vi "GetConfigure.vi"(8 "Error In":errorcluster, 11 "Keithley 6482 In":refnum<visa-resource-name>) -> (0 "Error Out":errorcluster, 2 "Configuration":string, 3 "Keithley 6482 Out":refnum<visa-resource-name>)   [LabVIEW 2014, in "Keithley-6482-Visa.lvlib"]
uses:
  Keithley-6482-Visa.lvlib
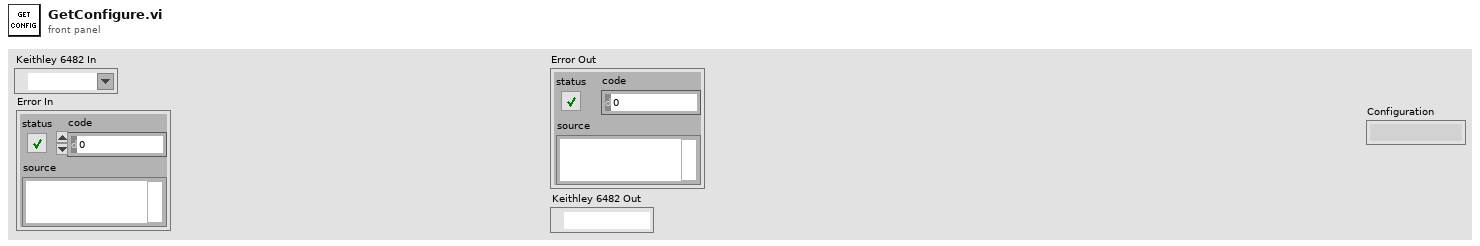
[diagram p1: front panel]
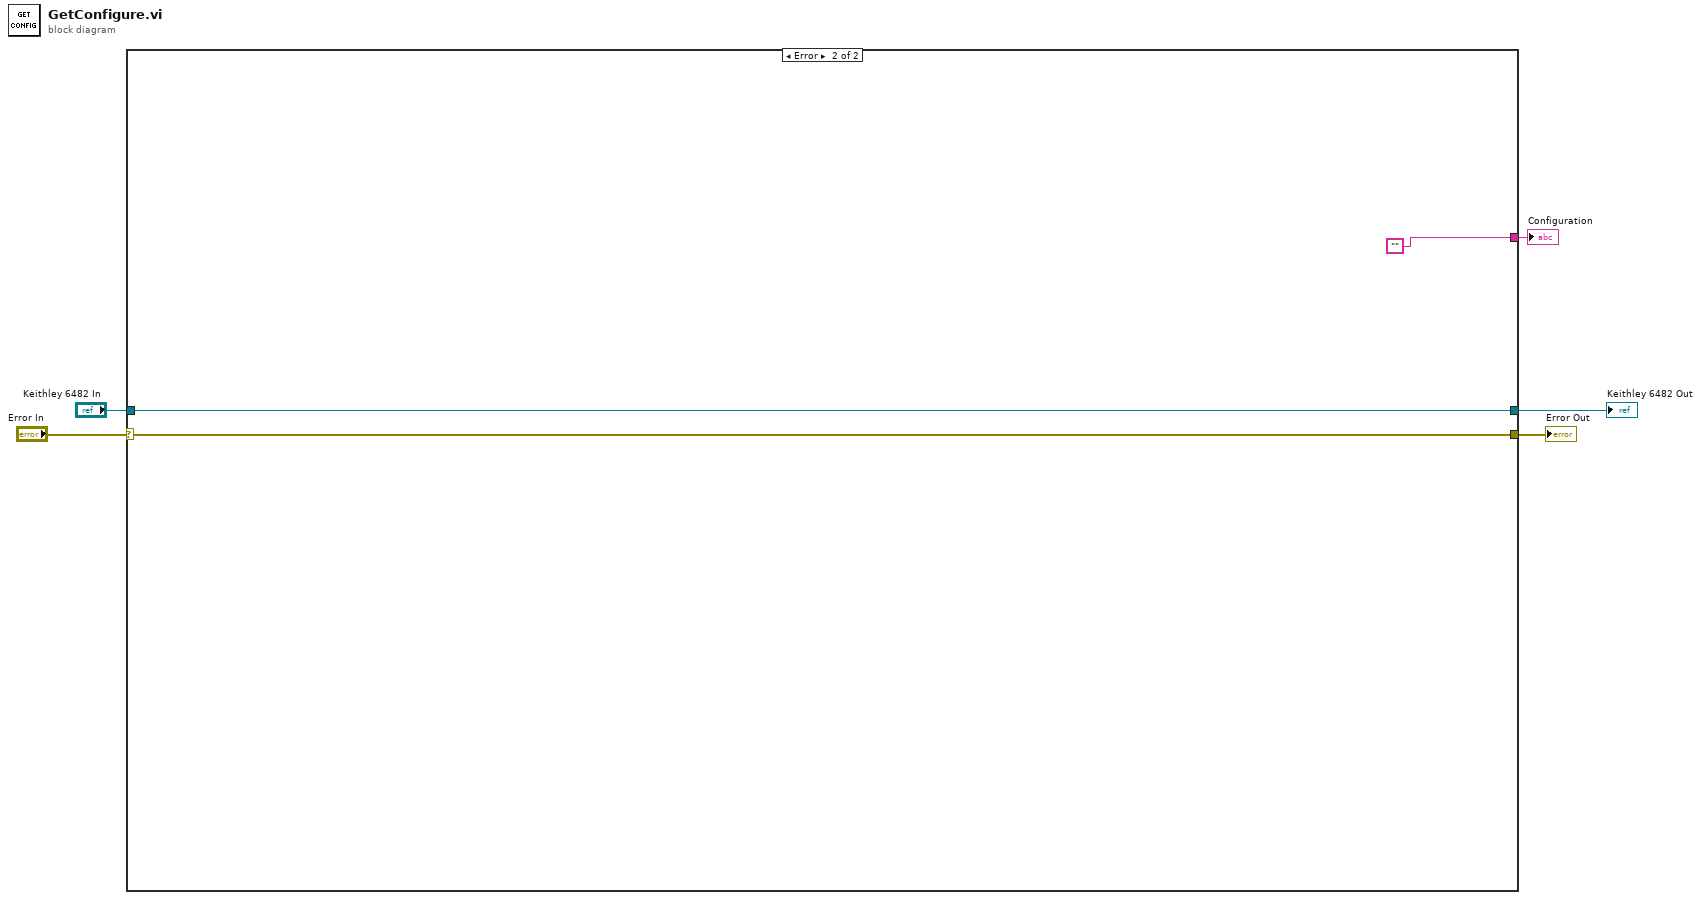
[diagram p0: block diagram]
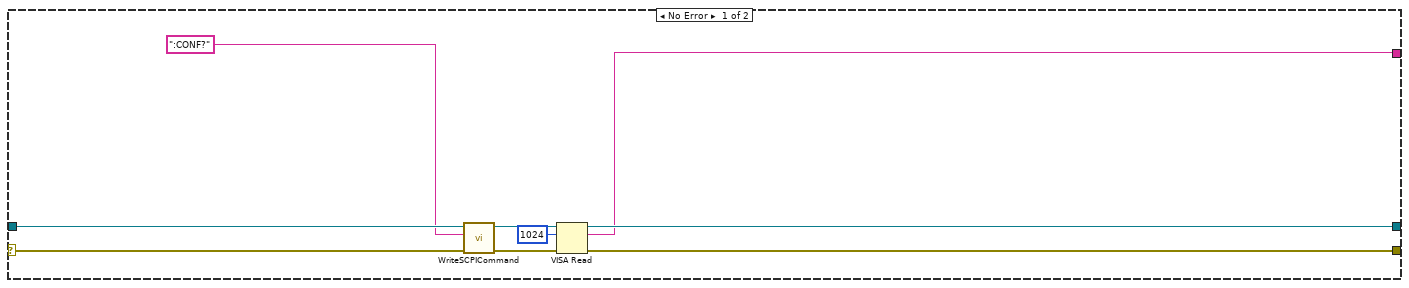
[diagram p2: hidden frame]
diagram:
  n1 = case shown="Error" "Error In" {
    selector: "Error In" -> [w14 w16]
    tunnel: "Keithley 6482 In" -> [w13 w17]
    tunnel: [w9 w16] -> w3
    tunnel: [w8 w17] -> w2
    tunnel: [w6 ""] -> w1
    frame No Error {
      n2 = call "WriteSCPICommand.vi"("Error In"=w14, "SCPI Command"=":CONF?" ("string"), "Keithley 6482 In"=w13) -> ("Error Out"=w10:errorcluster, "Keithley 6482 Out"=w11:refnum<visa-resource-name>)  [unwired: 7 in]
      n3 = VISA Read(VISA resource name=w11, byte count=u32 1024, error in (no error)=w10) -> (VISA resource name out=w8:refnum<visa-resource-name>, read buffer=w6:string, error out=w9:errorcluster)  [unwired: 1 out]
    }
    frame Error {
    }
  }
  "Error Out" <- w3
  "Keithley 6482 Out" <- w2
  "Configuration" <- w1
